vi "LoadProjectItemRecursively.vi"(8 "error in (no error)":errorcluster, 10 "ProjectItem In":refnum<vi>, 11 "Application in":refnum<vi>) -> (0 "error out":errorcluster, 3 "VIRefs":refnum<vi>[](array[refnum]))   [LabVIEW 2017]
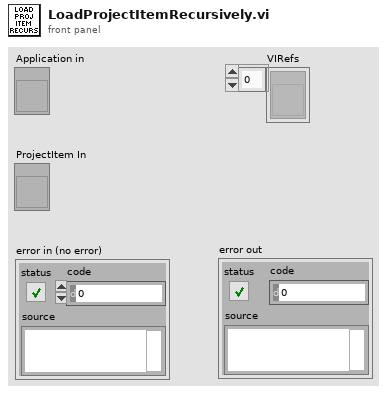
[diagram p1: front panel]
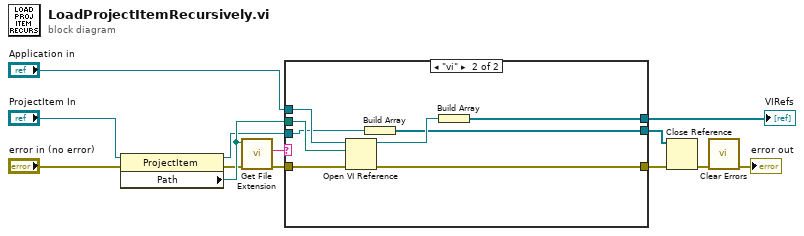
[diagram p0: block diagram]
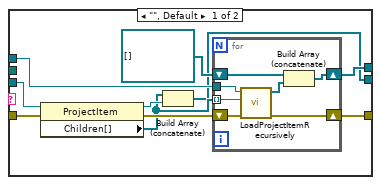
[diagram p2: hidden frame]
diagram:
  n1 = property class="ProjectItem"(reference="ProjectItem In", error in="error in (no error)") -> (reference out=w10:refnum<vi>, error out=w7:errorcluster, "Path"=w12:path)
  n2 = call <vilib>:"Get File Extension.vi"("error in (no error)"=w7, "file"=w12) -> ("error out"=w5:errorcluster, "lowercase file extension"=w11:string)  [unwired: 5 in, 3 out]
  n3 = case shown="\"vi\"" w11 {
    tunnel: "Application in" -> [w23 w38]
    tunnel: [w21 w35] -> w8
    tunnel: w12 -> [_ w37]
    tunnel: w10 -> [w22 w34]
    tunnel: w5 -> [w19 w32]
    tunnel: [w17 w31] -> w3
    tunnel: [w14 w33] -> w4
    frame "", Default {
      n4 = property class="ProjectItem"(reference=w22, error in=w19) -> (reference out=w16:refnum<vi>, error out=w18:errorcluster, "Children[]"=w15:refnum<vi>[])
      n5 = Build Array (concatenate)(w15, w16) -> (w14:refnum<vi>[])
      n6 = for {
        tunnel: w23 -> [w30]
        tunnel: w15 -> [w29] mode=indexing
        shift-right: [w26] -> w21
        shift-left: refnum<vi>[] [] ("VIRefs") -> [w28]
        shift-right: [w24] -> w17
        shift-left: w18 -> [w25]
        n7 = call "LoadProjectItemRecursively.vi"("error in (no error)"=w25, "ProjectItem In"=w29, "Application in"=w30) -> ("error out"=w24:errorcluster, "VIRefs"=w27:refnum<vi>[])  [unwired: 7 in]
        n8 = Build Array (concatenate)(w28, w27) -> (w26:refnum<vi>[])
      }
    }
    frame "vi" {
      n9 = Open VI Reference(application reference (local)=w38, vi path=w37, error in (no error)=w32) -> (vi reference=w36:refnum<vi>, error out=w31:errorcluster)  [unwired: 3 in]
      n10 = Build Array(w34) -> (w33:refnum<vi>[])
      n11 = Build Array(w36) -> (w35:refnum<vi>[])
    }
  }
  "VIRefs" <- w8
  n12 = Close Reference(reference=w4, error in (no error)=w3) -> (error out=w2:errorcluster)
  n13 = call <vilib>:"Clear Errors.vi"("error in (no error)"=w2) -> ("error out"=→"error out":errorcluster)  [unwired: 5 in, 1 out]
